vi "Initialize_Cluster_Points_Areas-1.vi"(1 "[IN] Number of frames":i32) -> (0 "[OUT] Cluster of \npoints and areas":T1(array[cluster]))   [LabVIEW 2017]
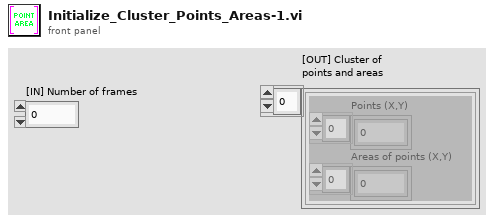
[diagram p1: front panel]
types:
  T1 = cluster{"Points (X,Y)":dbl[], "Areas of points (X,Y)":dbl[]}[]
  T2 = cluster{"Points (X,Y)":dbl[], "Areas of points (X,Y)":dbl[]}
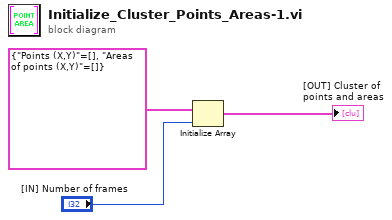
[diagram p0: block diagram]
diagram:
  n1 = Initialize Array(T2 {"Points (X,Y)"=[], "Areas of points (X,Y)"=[]}, "[IN] Number of frames") -> (→"[OUT] Cluster of \npoints and areas":T1)
